vi "LWXPS_DebugProfilerTimeUsageGet.vi"(0 "XPS Reference IN":refnum<k24>, 11 "LabVIEW error IN":errorcluster) -> (3 "XPS Reference OUT":refnum<k24>, 4 "Returned error code":i32, 6 "ISR Correct Profile Delta":dbl, 8 "ISR Groups Duration":dbl, 10 "ISR Init Param Duration":dbl, 14 "LabVIEW error OUT":errorcluster, 15 "XPS Error String":string)   [LabVIEW 2014]
uses:
  D:/XPSQ8_LabView_Library/Development/Source/Dll/Newport.XPS.CommandInterface.dll
  Dll/Newport.XPS.CommandInterface.dll
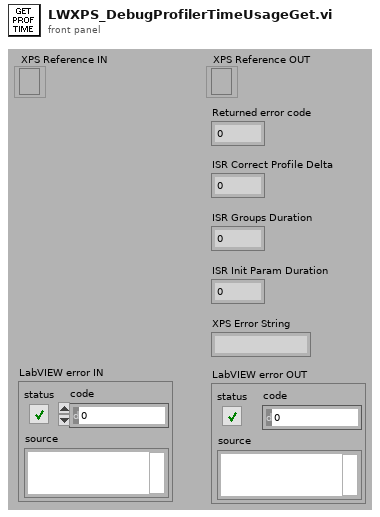
[diagram p1: front panel]
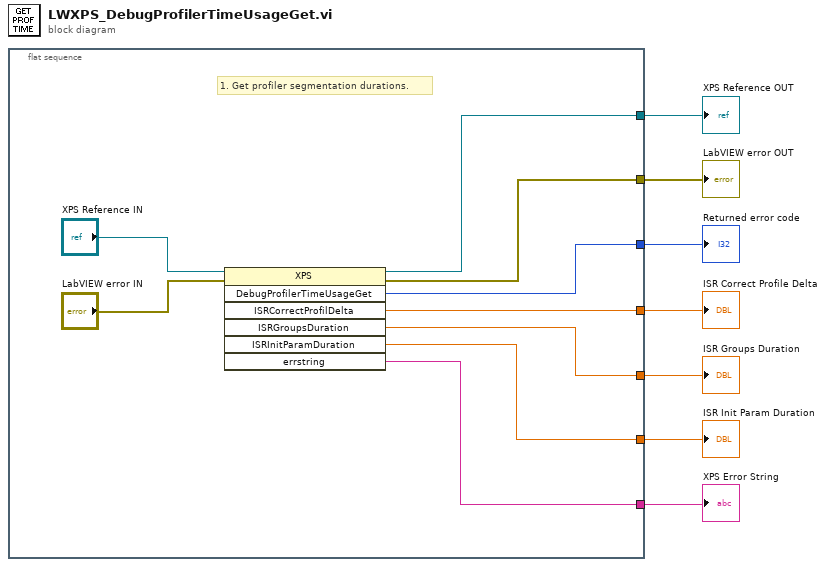
[diagram p0: block diagram]
diagram:
  n1 = flat-sequence {
    tunnel: [w14] -> w7
    tunnel: [w12] -> w6
    tunnel: [w15] -> w5
    tunnel: [w11] -> w2
    tunnel: [w10] -> w1
    tunnel: [w9] -> w3
    tunnel: [w8] -> w4
    frame #0 {
      # "1. Get profiler segmentation durations."
      n2 = invoke class="XPS" method="DebugProfilerTimeUsageGet"(reference="XPS Reference IN", error in="LabVIEW error IN") -> (reference out=w14:refnum<k24>, error out=w12:errorcluster, "DebugProfilerTimeUsageGet"=w15:i32, "ISRCorrectProfilDelta"=w9:dbl, "ISRGroupsDuration"=w11:dbl, "ISRInitParamDuration"=w10:dbl, "errstring"=w8:string)  [unwired: 5 in]
    }
  }
  "XPS Reference OUT" <- w7
  "LabVIEW error OUT" <- w6
  "Returned error code" <- w5
  "XPS Error String" <- w4
  "ISR Correct Profile Delta" <- w3
  "ISR Groups Duration" <- w2
  "ISR Init Param Duration" <- w1
